vi "image_transform_b&w&g.vi"(11 "Path":path) -> (3 "output array":u32[][](array[numeric]))   [LabVIEW 2015]
panel:
  out "8-bit pixmap":u8[][](array[numeric])
  out "24-bit pixmap":u32[][](array[numeric]) format="%x"
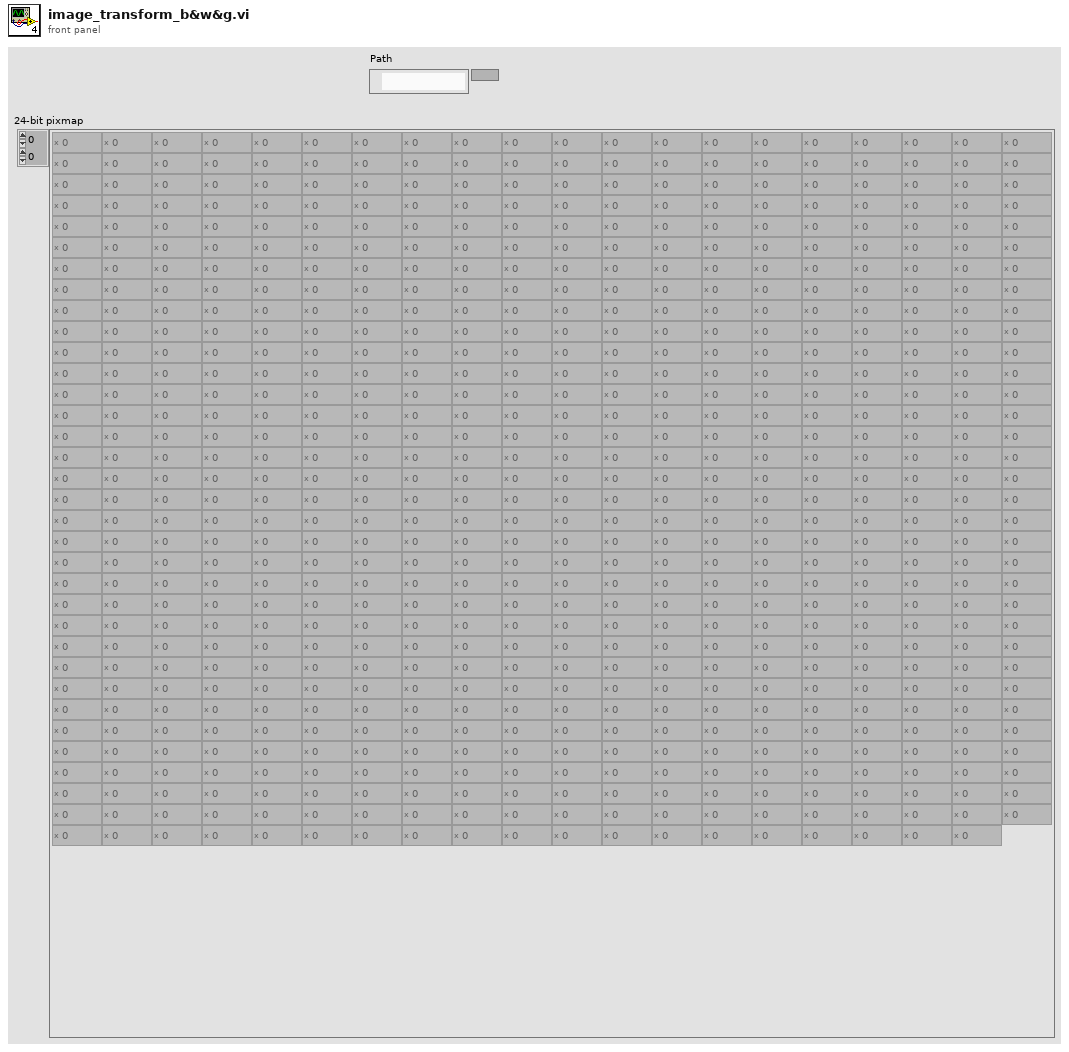
[diagram p1: front panel]
types:
  T1 = typedef "imagedata.ctl" = cluster{"image type":i32, "image depth":i32, "image":u8[], "mask":u8[], "colors":u32[], "Rectangle":cluster{"left":i16, "top":i16, "right":i16, "bottom":i16}}
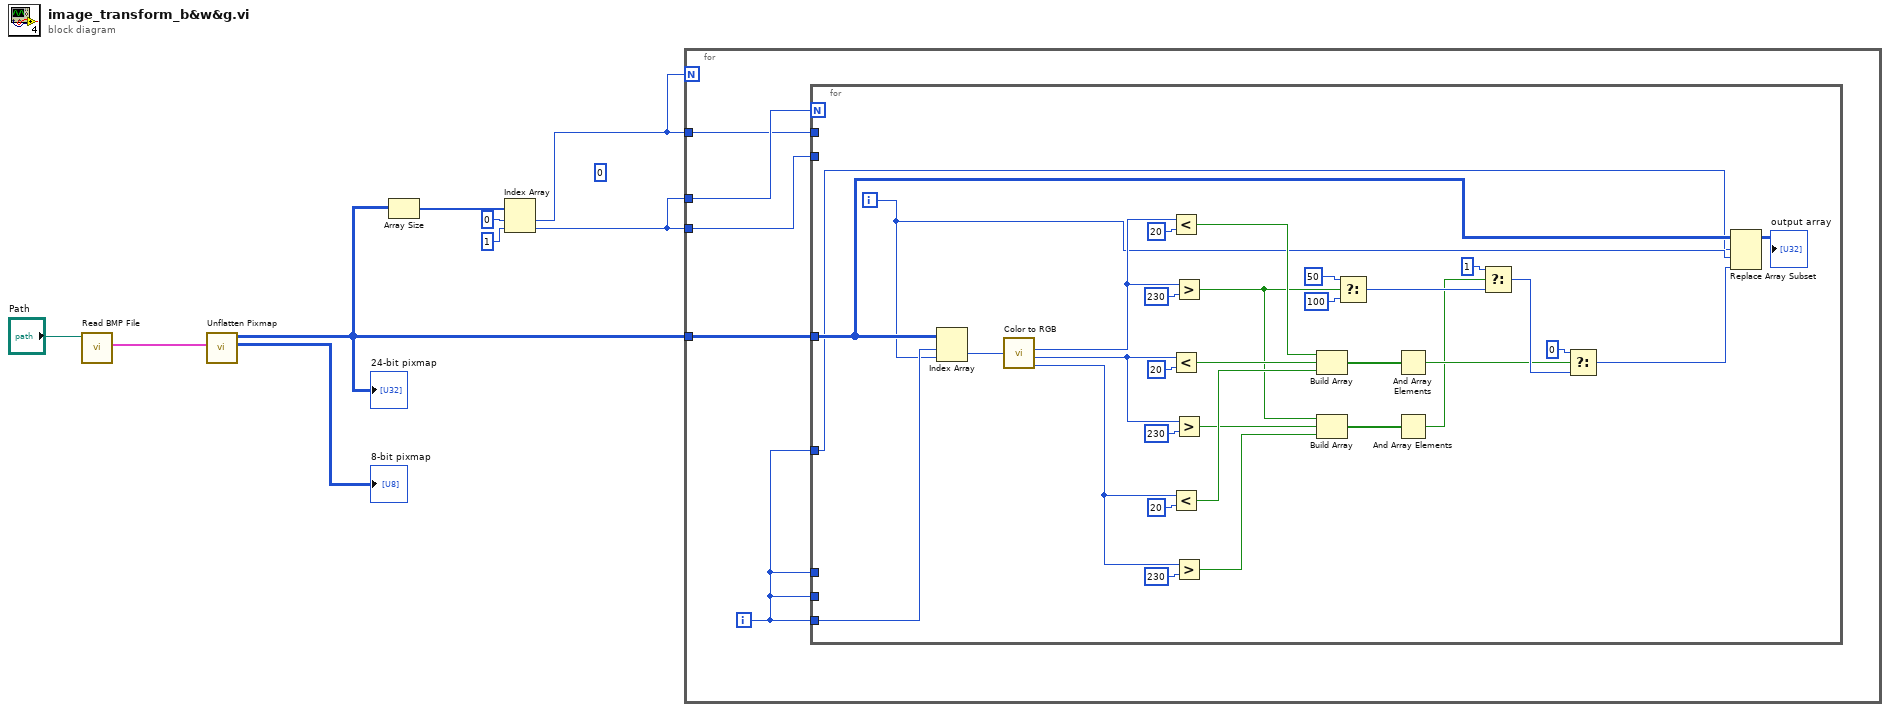
[diagram p0: block diagram]
diagram:
  (unwired) u8 0 ("element")
  n1 = call <vilib>:"Read BMP File.vi"("path to BMP file"="Path") -> ("image data"=w8:T1)  [unwired: 8 in, 2 out]
  n2 = call <vilib>:"Unflatten Pixmap.vi"("image data"=w8) -> ("8-bit pixmap"=→"8-bit pixmap":u8[][], "24-bit pixmap"=w4:u32[][])  [unwired: 4 in, 5 out]
  "24-bit pixmap" <- w4
  n3 = Array Size(array=w4) -> (size(s)=w7:i32[])
  n4 = Index Array(array=w7, index #1=0 ("index"), index #2=1 ("index")) -> (element #1=w2:i32, element #2=w1:i32)
  n5 = for {
    N: w2 -> [_]
    tunnel: w1 -> [w14]
    tunnel: w4 -> [w13]
    tunnel: w2 -> [w12]
    tunnel: w1 -> [w11]
    i -> [w10]
    n6 = for {
      N: w14 -> [_]
      tunnel: w13 -> [w19]
      tunnel: w10 -> [_]
      tunnel: w10 -> [w46]
      tunnel: w12 -> [_]
      tunnel: w11 -> [_]
      tunnel: w10 -> [_]
      tunnel: w10 -> [w17]
      i -> [w18]
      n7 = Index Array(array=w19, index (row)=w46, index (col)=w18) -> (element=w45:u32)
      n8 = call <vilib>:"Color to RGB.vi"("Color"=w45) -> ("R"=w38:u8, "G"=w37:u8, "B"=w36:u8)  [unwired: 1 out]
      n9 = Less?(x=w38, y=u8 20) -> (x < y?=w29:bool)
      n10 = Less?(x=w37, y=u8 20) -> (x < y?=w28:bool)
      n11 = Less?(x=w36, y=u8 20) -> (x < y?=w27:bool)
      n12 = Greater?(x=w38, y=u8 230) -> (0:w24:bool)
      n13 = Greater?(x=w37, y=u8 230) -> (0:w23:bool)
      n14 = Greater?(x=w36, y=u8 230) -> (0:w22:bool)
      n15 = Build Array(w29, w28, w27) -> (w26:bool[])
      n16 = Build Array(w24, w23, w22) -> (w21:bool[])
      n17 = Select(t=u32 50, s=w24, f=u32 100) -> (s? t:f=w30:u32)
      n18 = And Array Elements(Boolean array=w26) -> (logical AND=w25:bool)
      n19 = And Array Elements(Boolean array=w21) -> (logical AND=w20:bool)
      n20 = Select(t=u32 1, s=w20, f=w30) -> (s? t:f=w34:u32)
      n21 = Select(t=u32 0, s=w25, f=w34) -> (s? t:f=w16:u32)
      n22 = Replace Array Subset(array=w19, new element=w16, index (row)=w17, index (col)=w18) -> (→"output array":u32[][])
    }
  }
